vi "Signal Generator.vi"(1 "Signal Properties":T1={"Schedule"=enum."Constant", "Settings"=variant(dbl 0.0)}, 2 "Points":cluster{"X":dbl, "Y":dbl}[](array[cluster])) -> (0 "Signal":dbl[](array[numeric]))   [LabVIEW 2019]
uses:
  <vilib>/measure/NI_MABase.lvlib
  <vilib>/gmath/NI_Gmath.lvlib
  typedefs/Schedule Types/Schedule--Constant.ctl
  typedefs/Schedule Types/Schedule--Ramp.ctl
  typedefs/Schedule Types/Schedule--Function Generator.ctl
  typedefs/Schedule Types/Schedule--Formula.ctl
  Classes/Settings/ObjectSettings/ObjectSettings.lvclass
  typedefs/Schedule - enum.ctl
  typedefs/Voltage - cluster.ctl
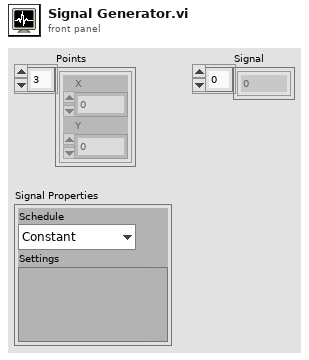
[diagram p1: front panel]
types:
  T1 = typedef "Voltage - cluster.ctl" = cluster{"Schedule":T2, "Settings":variant}
  T2 = typedef "Schedule - enum.ctl" = enum16{"Constant", "Ramp", "Fn. Generator", "Formula"}
  T3 = enum16{"Sine Wave", "Triangle Wave", "Square Wave", "Sawtooth Wave"}
  T4 = typedef "Schedule--Constant.ctl" = cluster{"Value":dbl}
  T5 = typedef "Schedule--Ramp.ctl" = cluster{"Start":dbl, "End":dbl}
  T6 = typedef "Schedule--Function Generator.ctl" = cluster{"Min Value":dbl, "Max Value":dbl, "Duty Cycle (%)":dbl, "Signal Type":u16, "Cycle Number":dbl, "Phase (degrees)":dbl}
  T7 = typedef "Schedule--Formula.ctl" = cluster{"formula":string, "formula length (nm)":dbl, "formula resolution (nm)":dbl}
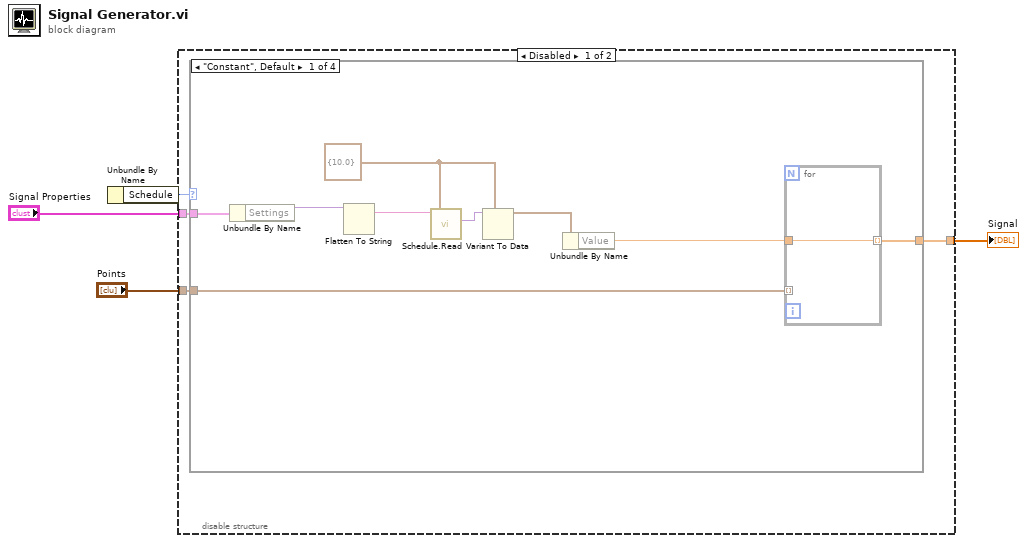
[diagram p0: block diagram]
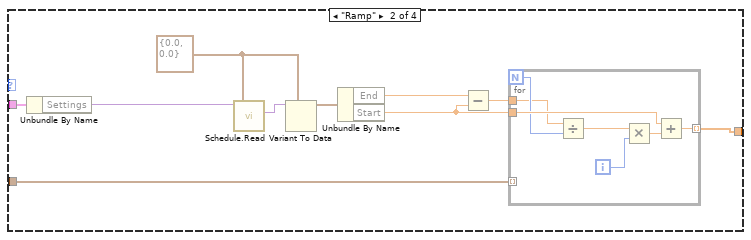
[diagram p2: hidden frame]
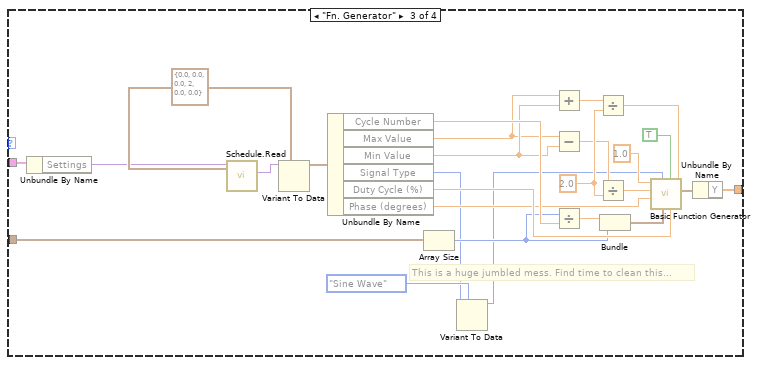
[diagram p3: hidden frame]
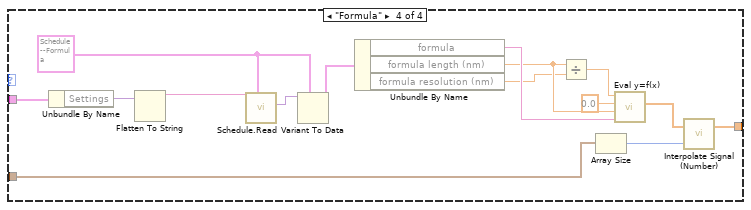
[diagram p4: hidden frame]
diagram:
  n1 = disable-structure shown="Disabled" {
    disable-tunnel: [w7 _] -> w3
    disable-tunnel: "Signal Properties" -> [w5 _]
    disable-tunnel: "Points" -> [w4 _]
    frame Disabled {
      n2 = Unbundle By Name(w5) -> ("Schedule"=w6:T2)
      n3 = case shown="\"Constant\", Default" w6 {
        tunnel: w5 -> [w13 w22 w42 w67]
        tunnel: w4 -> [w16 w27 w48 w66]
        tunnel: [w14 w24 w60 w71] -> w7
        frame "Constant", Default {
          w11 = T4 {"Value"=10.0} ("Constant")
          n4 = Unbundle By Name(w13) -> ("Settings"=w8:variant)
          n5 = Flatten To String(anything=w8) -> (data string=w9:string)  [unwired: 3 in, 2 out]
          n6 = call "Schedule.Read.vi"("Data to Read"=w11, "Schedule <JSON> In"=w9) -> ("Data Out"=w10:variant)  [unwired: 7 in, 2 out]
          n7 = Variant To Data(type=w11, Variant=w10) -> (data=w12:T4)  [unwired: 1 in, 1 out]
          n8 = Unbundle By Name(w12) -> ("Value"=w15:dbl)
          n9 = for {
            tunnel: w16 -> [_] mode=indexing
            tunnel: w15 -> [w17]
            tunnel: [w17] -> w14 mode=indexing
          }
        }
        frame "Ramp" {
          w20 = T5 {"Start"=0.0, "End"=0.0} ("Ramp")
          n10 = Unbundle By Name(w22) -> ("Settings"=w21:variant)
          n11 = call "Schedule.Read.vi"("Data to Read"=w20, "Schedule <JSON> In"=w21) -> ("Data Out"=w18:variant)  [unwired: 7 in, 2 out]
          n12 = Variant To Data(type=w20, Variant=w18) -> (data=w19:T5)  [unwired: 1 in, 1 out]
          n13 = Unbundle By Name(w19) -> ("End"=w26:dbl, "Start"=w23:dbl)
          n14 = Subtract(x=w26, y=w23) -> (x-y=w25:dbl)
          n15 = for {
            N -> [w29]
            tunnel: w27 -> [_] mode=indexing
            tunnel: w25 -> [w28]
            tunnel: w23 -> [w32]
            tunnel: [w31] -> w24 mode=indexing
            i -> [w34]
            n16 = Divide(x=w28, y=w29) -> (x/y=w30:dbl)
            n17 = Multiply(x=w30, y=w34) -> (x*y=w33:dbl)
            n18 = Add(x=w32, y=w33) -> (x+y=w31:dbl)
          }
        }
        frame "Fn. Generator" {
          w41 = T6 {"Min Value"=0.0, "Max Value"=0.0, "Duty Cycle (%)"=0.0, "Signal Type"=2, "Cycle Number"=0.0, "Phase (degrees)"=0.0} ("Fn. Gen")
          w55 = 2.0 ("y")
          # "This is a huge jumbled mess. Find time to clean this..."
          n19 = Unbundle By Name(w42) -> ("Settings"=w40:variant)
          n20 = call "Schedule.Read.vi"("Data to Read"=w41, "Schedule <JSON> In"=w40) -> ("Data Out"=w38:variant)  [unwired: 7 in, 2 out]
          n21 = Variant To Data(type=w41, Variant=w38) -> (data=w39:T6)  [unwired: 1 in, 1 out]
          n22 = Unbundle By Name(w39) -> ("Cycle Number"=w58:dbl, "Max Value"=w53:dbl, "Min Value"=w54:dbl, "Signal Type"=w36:u16, "Duty Cycle (%)"=w57:dbl, "Phase (degrees)"=w49:dbl)
          n23 = Array Size(array=w48) -> (size(s)=w44:i32)
          n24 = Variant To Data(type=T3."Sine Wave" ("signal type"), Variant=w36) -> (data=w35:T3)  [unwired: 1 in, 1 out]
          n25 = Add(x=w53, y=w54) -> (x+y=w52:dbl)
          n26 = Subtract(x=w53, y=w54) -> (x-y=w45:dbl)
          n27 = Divide(x=w44, y=w58) -> (x/y=w59:dbl)
          n28 = Divide(x=w52, y=w55) -> (x/y=w46:dbl)
          n29 = Divide(x=w45, y=w55) -> (x/y=w56:dbl)
          n30 = Bundle(w59, w44) -> (w47:cluster{dbl, i32})  [unwired: 1 in]
          n31 = call <vilib>:"Basic Function Generator.vi"("offset"=w46, "square wave duty cycle (%)"=w57, "reset signal"=TRUE, "sampling info"=w47, "signal type"=w35, "phase"=w49, "amplitude"=w56, "frequency"=1.0) -> ("signal out"=w50:waveform(dbl))  [unwired: 1 in, 2 out]
          n32 = Unbundle By Name(w50) -> ("Y"=w60:dbl[])
        }
        frame "Formula" {
          w65 = T7 {"formula"="1*(step(170-t)*cos(0.62831853071*t)+step(t-170)*cos(0.62831853071*(t-170))*(-1))", "formula length (nm)"=340.0, "formula resolution (nm)"=0.001} ("Formula")
          n33 = Unbundle By Name(w67) -> ("Settings"=w62:variant)
          n34 = Flatten To String(anything=w62) -> (data string=w61:string)  [unwired: 3 in, 2 out]
          n35 = call "Schedule.Read.vi"("Data to Read"=w65, "Schedule <JSON> In"=w61) -> ("Data Out"=w63:variant)  [unwired: 7 in, 2 out]
          n36 = Variant To Data(type=w65, Variant=w63) -> (data=w64:T7)  [unwired: 1 in, 1 out]
          n37 = Unbundle By Name(w64) -> ("formula"=w74:string, "formula length (nm)"=w69:dbl, "formula resolution (nm)"=w68:dbl)
          n38 = Divide(x=w69, y=w68) -> (x/y=w73:dbl)
          n39 = Array Size(array=w66) -> (size(s)=w70:i32)
          n40 = call <vilib>:"Eval y=f(x).vi"("formula"=w74, "end"=w69, "start"=0.0, "number of points"=w73) -> ("Y Values"=w72:dbl[])  [unwired: 3 out]
          n41 = call "Interpolate Signal (Number).vi"("desired # of points"=w70, "Array"=w72) -> ("Resampled Array"=w71:dbl[])  [unwired: 1 in]
        }
      }
    }
    frame Enabled {
    }
  }
  "Signal" <- w3
